vi "mono-lambda.vi"(8 "Error In":errorcluster, 10 "set":bool, 11 "Monochromator":refnum<vi>) -> (0 "Error Out":errorcluster)   [LabVIEW 2016]
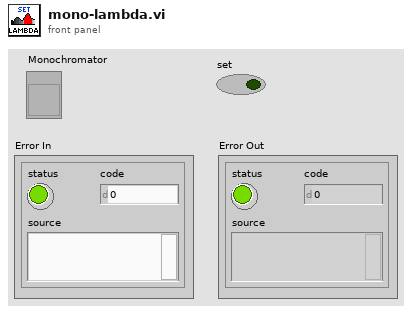
[diagram p1: front panel]
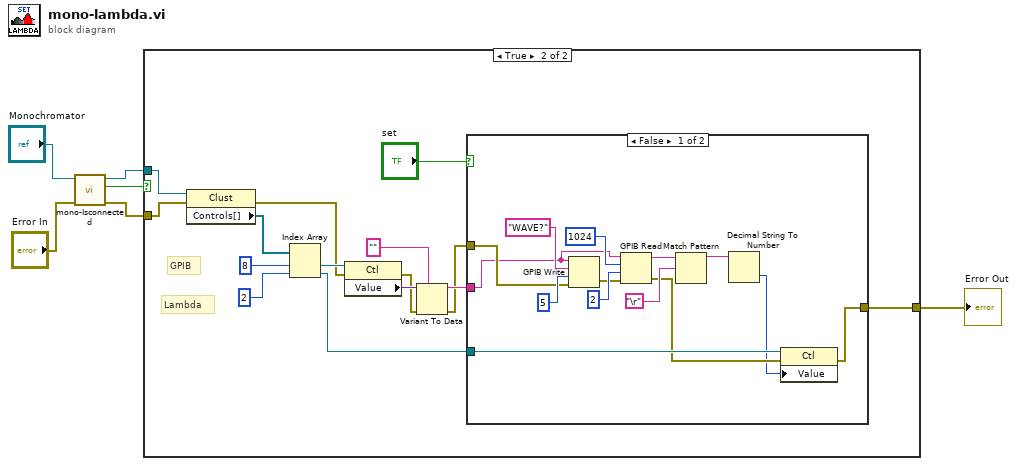
[diagram p0: block diagram]
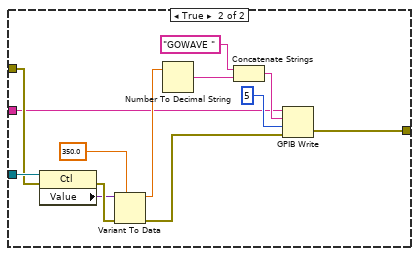
[diagram p3: hidden frame]
diagram:
  n1 = call "mono-Isconnected.vi"("error in (no error)"="Error In", "Monochromator"="Monochromator") -> ("error out"=w1:errorcluster, "Connected"=w3:bool, "Monochromator out"=w2:refnum<vi>)  [unwired: 7 in]
  n2 = case shown="True" w3 {
    tunnel: [w7 w8] -> w4
    tunnel: w2 -> [_ w18]
    tunnel: w1 -> [w7 w17]
    frame False {
    }
    frame True {
      # "Lambda"
      # "GPIB"
      n3 = property class="Clust"(reference=w18, error in=w17) -> (error out=w15:errorcluster, "Controls[]"=w21:refnum<vi>[])  [unwired: 1 out]
      n4 = Index Array(array=w21, index #1=8 ("index"), index #2=2 ("index")) -> (element #1=w16:refnum<vi>, element #2=w11:refnum<vi>)
      n5 = property class="Ctl"(reference=w16, error in=w15) -> (error out=w12:errorcluster, "Value"=w14:variant)  [unwired: 1 out]
      n6 = Variant To Data(error in=w12, type="", Variant=w14) -> (data=w10:string, error out=w9:errorcluster)
      n7 = case shown="False" "set" {
        tunnel: w11 -> [w27 w45]
        tunnel: w10 -> [w23 w39]
        tunnel: w9 -> [w31 w44]
        tunnel: [w24 w37] -> w8
        frame False {
          n8 = GPIB Write(0:w23, 1:"WAVE?" ("data"), 2:i16 5 ("mode (0)"), 3:w31) -> (6:w34:errorcluster)  [unwired: 1 in, 1 out]
          n9 = GPIB Read(0:w23, 1:1024 ("byte count"), 2:i16 2 ("mode (0)"), 3:w34) -> (5:w29:string, 7:w26:errorcluster)  [unwired: 1 in, 1 out]
          n10 = Match Pattern(string=w29, regular expression="\r") -> (before substring=w30:string)  [unwired: 1 in, 3 out]
          n11 = Decimal String To Number(string=w30) -> (number=w25:i32)  [unwired: 2 in, 1 out]
          n12 = property class="Ctl"(reference=w27, error in=w26, "Value"=w25) -> (error out=w24:errorcluster)  [unwired: 1 out]
        }
        frame True {
          n13 = property class="Ctl"(reference=w45, error in=w44) -> (error out=w43:errorcluster, "Value"=w42:variant)  [unwired: 1 out]
          n14 = Variant To Data(error in=w43, type=350.0 ("Lambda"), Variant=w42) -> (data=w40:dbl, error out=w38:errorcluster)
          n15 = Number To Decimal String(number=w40) -> (decimal integer string=w47:string)  [unwired: 1 in]
          n16 = Concatenate Strings("GOWAVE ", w47) -> (w48:string)
          n17 = GPIB Write(0:w39, 1:w48, 2:i16 5 ("mode (0)"), 3:w38) -> (6:w37:errorcluster)  [unwired: 1 in, 1 out]
        }
      }
    }
  }
  "Error Out" <- w4
